vi "Controle_ATM.vi"(11 "seconds to wait":u32) -> (0 "String 2":string, 3 "Atm":bool)   [LabVIEW 2011]
uses:
  <vilib>/DAQmx/write.llb/DAQmx Write (Digital Bool 1Line 1Point).vi
  <vilib>/DAQmx/create/channels.llb/DAQmx Create Channel (DO-Digital Output).vi
  <vilib>/DAQmx/miscellaneous.llb/DAQmx Fill In Error Info.vi
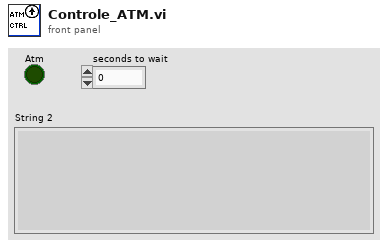
[diagram p1: front panel]
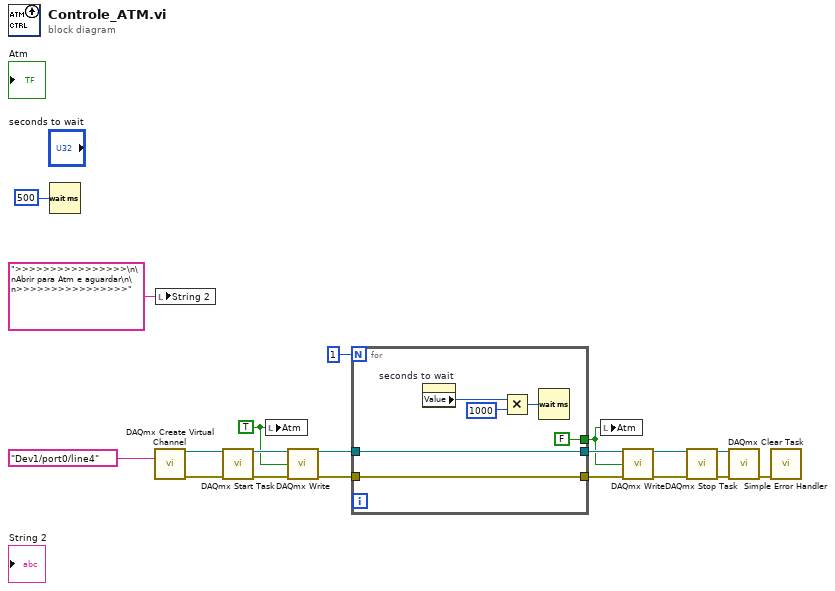
[diagram p0: block diagram]
diagram:
  w9 = TRUE ("Boolean")
  n1 = Wait (ms)(milliseconds to wait=u32 500) -> ()  [unwired: 1 out]
  n2 = call-poly <vilib>:"DAQmx Create Virtual Channel.vi"("lines"=tag "Dev1/port0/line4") -> ("task out"=w18:refnum<k21>, "error out"=w17:errorcluster)  [unwired: 13 in]
  n3 = local write "String 2"(">>>>>>>>>>>>>>>>\n\nAbrir para Atm e aguardar\n\n>>>>>>>>>>>>>>>>" ("String")) -> ()
  n4 = call <vilib>:"DAQmx Start Task.vi"("task/channels in"=w18, "error in"=w17) -> ("task out"=w16:refnum<k21>, "error out"=w15:errorcluster)  [unwired: 12 in]
  n5 = local write "Atm"(w9) -> ()
  n6 = call-poly <vilib>:"DAQmx Write.vi"("task/channels in"=w16, "data"=w9, "error in"=w15) -> ("task out"=w6:refnum<k21>, "error out"=w4:errorcluster)  [unwired: 10 in, 1 out]
  n7 = for {
    N: 1 -> [_]
    tunnel: w6 -> [w25]
    tunnel: [w25] -> w5
    tunnel: w4 -> [w24]
    tunnel: [w24] -> w3
    tunnel: [FALSE ("Boolean")] -> w1
    n8 = property on="seconds to wait" class="DigNum (strict)"() -> ("Value"=w21:u32)  [unwired: 2 in, 2 out]
    n9 = Multiply(x=w21, y=u32 1000) -> (x*y=w22:u32)
    n10 = Wait (ms)(milliseconds to wait=w22) -> ()  [unwired: 1 out]
  }
  n11 = local write "Atm"(w1) -> ()
  n12 = call-poly <vilib>:"DAQmx Write.vi"("task/channels in"=w5, "data"=w1, "error in"=w3) -> ("task out"=w11:refnum<k21>, "error out"=w12:errorcluster)  [unwired: 10 in, 1 out]
  n13 = call <vilib>:"DAQmx Stop Task.vi"("task/channels in"=w11, "error in"=w12) -> ("task out"=w13:refnum<k21>, "error out"=w14:errorcluster)  [unwired: 12 in]
  n14 = call <vilib>:"DAQmx Clear Task.vi"("task in"=w13, "error in"=w14) -> ("error out"=w19:errorcluster)  [unwired: 13 in]
  n15 = call <vilib>:"Simple Error Handler.vi"("error in (no error)"=w19) -> ()  [unwired: 4 in, 5 out]
